vi "Simple Solenoid.vi"(1 "Value to Write 2":bool, 2 "Value to Write":bool) -> ()   [LabVIEW 2018]
doc: "Simple Solenoid Example\n\nThis example shows how to set the value of a Solenoid Channel.\n\nIt works with the PCM (Pneumatic Control Module) communicating with the roboRIO over CAN bus. The PCM must also be supplied with 12V DC from the PDP (Power Distribution Panel).\n\nThe Compressor, Pressure Switch, and Solenoid are all wired to the PCM \n\nThis example expects a USB cable connected from your development PC to the Type B USB Jack (next to the power input) on the roboRIO.\n\nThis example expects the Driver Station to be running."
uses:
  <vilib>/Rock Robotics/WPI/Solenoid/WPI_SolenoidValue.ctl
  <vilib>/Rock Robotics/WPI/Solenoid/WPI_SolenoidSetEnum.vi
panel:
  in  "stop 2":bool
  in  "stop":bool
  # "Set this input before running."
  # "This can be set while running."
  # "On"
  # "Off"
  # "Wiring Diagram"
  # "Pneumatic Control Module"
  # "To Solenoid"
  # "CAN"
  # "COMPRESSOR OUT"
  # "PRESSURE"
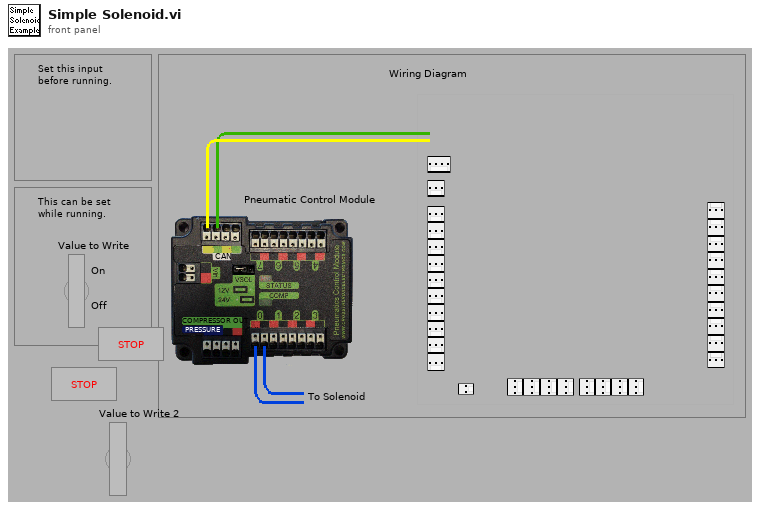
[diagram p1: front panel]
types:
  T1 = typedef "WPI_SolenoidDevRef.ctl" = cluster{"DevStatus":errorcluster, "Pneumatics Control Module":u8, "Forward Solenoid Channel":T2, "Reverse Solenoid Channel":T2}
  T2 = typedef "WPI_SolenoidChannel.ctl" = enum8{"Solenoid 0", "Solenoid 1", "Solenoid 2", "Solenoid 3", "Solenoid 4", "Solenoid 5", "Solenoid 6", "Solenoid 7", "Invalid"}
  T3 = typedef "WPI_SolenoidValue.ctl" = enum16{"Off", "On", "Forward", "Reverse"}
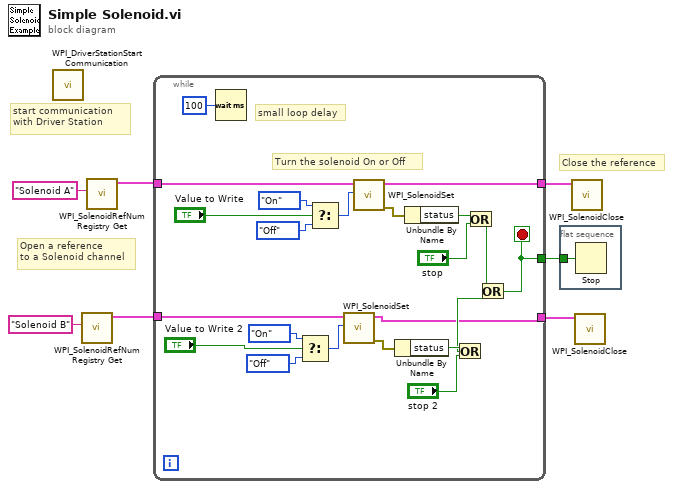
[diagram p0: block diagram]
diagram:
  # "start communication with Driver Station"
  # "Close the reference"
  # "Open a reference \nto a Solenoid channel"
  n1 = call <vilib>:"WPI_DriverStationStart Communication.vi"() -> ()  [unwired: 2 in, 10 out]
  n2 = call <vilib>:"WPI_SolenoidRefNum Registry Get.vi"("refnum name"="Solenoid B") -> ("SolenoidDevRef"=w1:T1)  [unwired: 9 in, 1 out]
  n3 = call <vilib>:"WPI_SolenoidRefNum Registry Get.vi"("refnum name"="Solenoid A") -> ("SolenoidDevRef"=w4:T1)  [unwired: 9 in, 1 out]
  n4 = while {
    tunnel: w4 -> [w28]
    tunnel: [w27] -> w7
    tunnel: [w10] -> w6
    tunnel: w1 -> [w9]
    tunnel: [w8] -> w3
    stop <- w10 stop-if-true
    # "small loop delay"
    # "Turn the solenoid On or Off"
    n5 = Wait (ms)(milliseconds to wait=u32 100) -> ()  [unwired: 1 out]
    n6 = Select(t=WPI_SolenoidValue."On" ("Value"), s="Value to Write 2", f=WPI_SolenoidValue."Off" ("Value")) -> (s? t:f=w13:T3)
    n7 = Select(t=WPI_SolenoidValue."On" ("Value"), s="Value to Write", f=WPI_SolenoidValue."Off" ("Value")) -> (s? t:f=w20:T3)
    n8 = call-poly <vilib>:"WPI_SolenoidSet.vi"("Value"=w13, "SolenoidDevRef"=w9) -> ("error out"=w19:errorcluster, "SolenoidDevRef"=w8:T1)  [unwired: 1 in, 7 out]
    n9 = call-poly <vilib>:"WPI_SolenoidSet.vi"("Value"=w20, "SolenoidDevRef"=w28) -> ("error out"=w26:errorcluster, "SolenoidDevRef"=w27:T1)  [unwired: 1 in, 7 out]
    n10 = Unbundle By Name(w19) -> ("status"=w18:bool)
    n11 = Unbundle By Name(w26) -> ("status"=w25:bool)
    n12 = Or(x=w18, y="stop 2") -> (x .or. y?=w12:bool)
    n13 = Or(x=w25, y="stop") -> (x .or. y?=w11:bool)
    n14 = Or(x=w11, y=w12) -> (x .or. y?=w10:bool)
  }
  n15 = flat-sequence {
    tunnel: w6 -> [w30]
    frame #0 {
      n16 = Stop(stop? (T)=w30) -> ()
    }
  }
  n17 = call <vilib>:"WPI_SolenoidClose.vi"("SolenoidDevRef"=w7) -> ()  [unwired: 1 in, 10 out]
  n18 = call <vilib>:"WPI_SolenoidClose.vi"("SolenoidDevRef"=w3) -> ()  [unwired: 1 in, 10 out]
